vi "手指.vi"(0 "指中":path, 3 "指尖":path) -> (6 "手指":refnum<vi>, 7 "指尖":refnum<vi>)   [LabVIEW 2016]
uses:
  <vilib>/picture/3D Picture Control/NI_3D Picture Control.lvlib
panel:
  out "机械手":refnum<vi>(3d-picture)
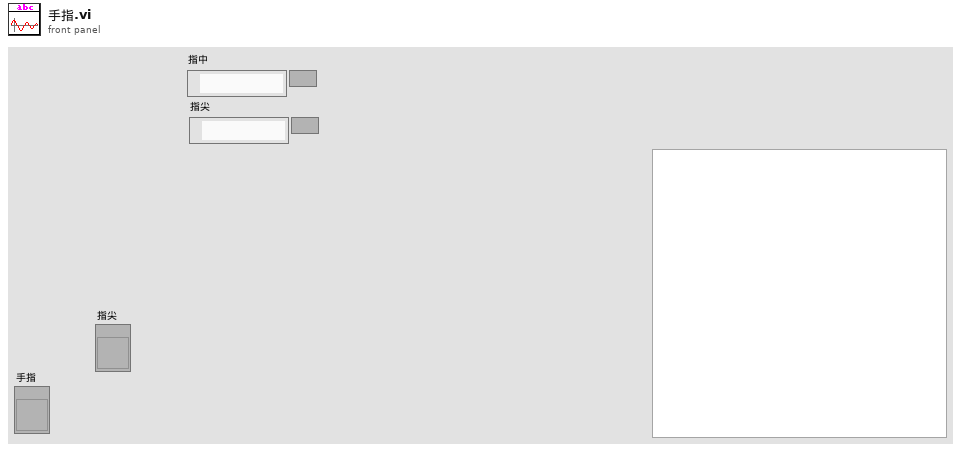
[diagram p1: front panel]
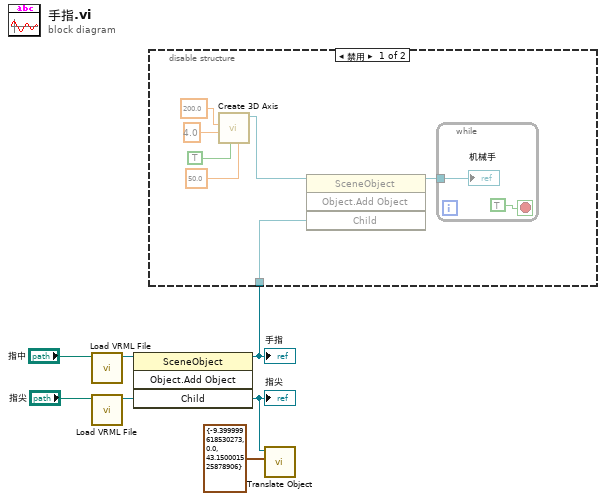
[diagram p0: block diagram]
diagram:
  n1 = call <vilib>:"Load VRML File.vi"("Path"="指中") -> ("Scene:Read Scene File"=w5:refnum<vi>)  [unwired: 9 in, 1 out]
  n2 = call <vilib>:"Load VRML File.vi"("Path"="指尖") -> ("Scene:Read Scene File"=w7:refnum<vi>)  [unwired: 9 in, 1 out]
  n3 = invoke class="SceneObject" method="Object.Add Object"(reference=w5, "Child"=w7) -> (reference out=w3:refnum<vi>, "Child"=w4:refnum<vi>)  [unwired: 2 in, 2 out]
  "手指" <- w3
  "指尖" <- w4
  n4 = disable-structure shown="禁用" {
    disable-tunnel: w3 -> [w9 _]
    frame Disabled {
      n5 = call <vilib>:"Create 3D Axis.vi"("Character Size"=sgl 50.0, "Axis label?"=TRUE, "Radius"=sgl 4.0, "Length"=sgl 200.0) -> ("New Object Refnum"=w10:refnum<vi>)  [unwired: 6 in, 1 out]
      n6 = invoke class="SceneObject" method="Object.Add Object"(reference=w10, "Child"=w9) -> (reference out=w8:refnum<vi>)  [unwired: 2 in, 3 out]
      n7 = while {
        tunnel: w8 -> [w16]
        stop <- TRUE ("停止") stop-if-true
        "机械手" <- w16
      }
    }
    frame Enabled {
    }
  }
  n8 = call <vilib>:"Translate Object.vi"("Translation"=cluster{"X":sgl, "Y":sgl, "Z":sgl} {"X"=-9.4, "Y"=0.0, "Z"=43.15}, "Scene.Object In"=w4) -> ()  [unwired: 8 in, 2 out]
